vi "Get Key Line.vi"(10 "key description":string, 11 "info data":string) -> (2 "key found?":bool, 3 "key value":string)   [LabVIEW 2013, in "infolib.lvlib"]
doc: "Finds a line starting with a <b>key description</b> in string <b>info data</b> and return value of the key. If the key is found, output <b>key found?</b> is true even if the value of the key is empty."
uses:
  infolib.lvlib
  <vilib>/regexp/Match Regular Expression.xnode
panel:
  # "testing string:"
  # "test1 :: 1\ntest2 :: 22\n#startsection:: 1\nAAA\n#startsection:: 2\nBBB\n\t  \t#endsection:: 2\nCCC\n#endsection:: 1\ntest3::333\n   test4:: 4444\n#startsection:: X\nDDD\n#endsection:: X\ntest5"
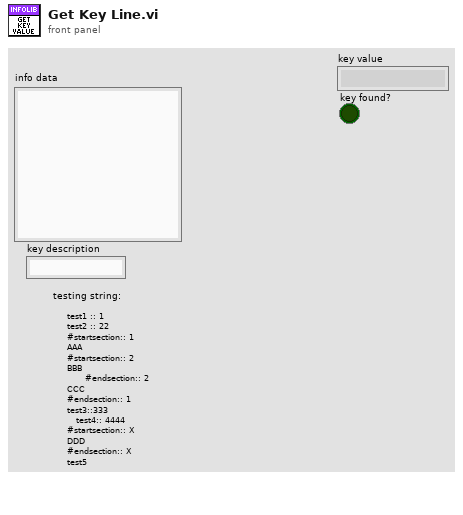
[diagram p1: front panel]
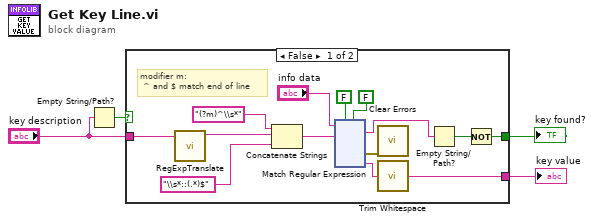
[diagram p0: block diagram]
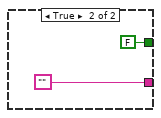
[diagram p2: hidden frame]
diagram:
  n1 = Empty String/Path?(string/path="key description") -> (empty?=w2:bool)
  n2 = case shown="False" w2 {
    tunnel: [w8 ""] -> w4
    tunnel: "key description" -> [w12 _]
    tunnel: [w6 FALSE] -> w1
    frame False {
      # "modifier m:\n ^ and $ match end of line"
      n3 = call "RegExpTranslate.vi"("string"=w12) -> ("regexp safe string"=w11:string)  [unwired: 10 in]
      n4 = Concatenate Strings("(?m)^\\s*" ("section name"), w11, "\\s*::(.*)$" ("section name")) -> (w13:string)
      n5 = xnode "Match Regular Expression"("input string"="info data", "regular expression"=w13, "ignore case? (F)"=FALSE, "multiline? (F)"=FALSE) -> ("whole match"=w5:string, "error out"=w17:errorcluster, "submatch 1"=w16:string)  [unwired: 2 in, 3 out]
      n6 = call <vilib>:"Clear Errors.vi"("error in (no error)"=w17) -> ()  [unwired: 6 in, 1 out]
      n7 = call <vilib>:"Trim Whitespace.vi"("string"=w16) -> ("trimmed string"=w8:string)  [unwired: 1 in]
      n8 = Empty String/Path?(string/path=w5) -> (empty?=w7:bool)
      n9 = Not(x=w7) -> (.not. x?=w6:bool)
    }
    frame True {
    }
  }
  "key value" <- w4
  "key found?" <- w1
